vi "test Flush.vi"(8 "error in (no error)":errorcluster, 11 "TestCase in":refnum<class "Message Queue Test Case.lvclass">) -> (0 "error out":errorcluster, 3 "TestCase out":refnum<class "Message Queue Test Case.lvclass">)   [LabVIEW 2017, in "Message Queue Test Case.lvclass"]
uses:
  Message Queue Test Case.lvclass
  Message Queue Test Case.lvclass/Message Queue Test Case.ctl
  Message/Abstract Message/Abstract Message.lvclass
  Message Queue/Abstract Message Queue/Abstract Message Queue.lvclass
  <vilib>/addons/_JKI Toolkits/VI Tester/TestCase.llb/TestCase.lvclass
  C:/Program Files (x86)/National Instruments/LabVIEW 2017/vi.lib/addons/_JKI Toolkits/VI Tester/TestCase.llb/TestCase.lvclass
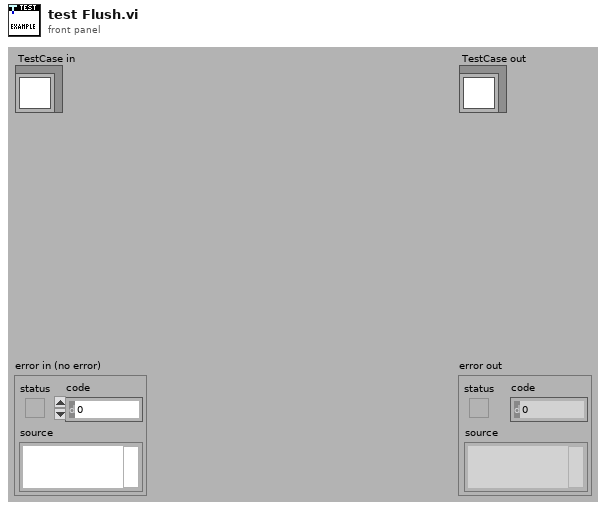
[diagram p1: front panel]
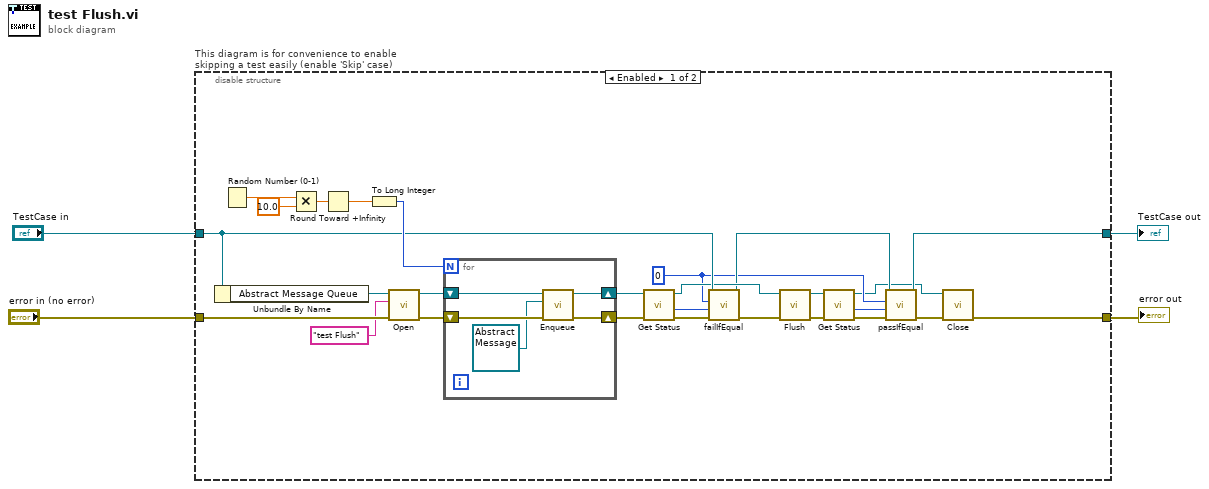
[diagram p0: block diagram]
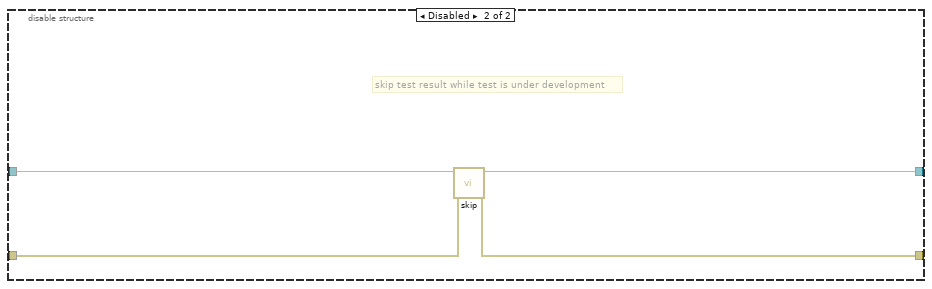
[diagram p2: hidden frame]
diagram:
  n1 = disable-structure "This diagram is for convenience to enable skipping a test easily (enable 'Skip' case)" shown="Enabled" {
    disable-tunnel: "TestCase in" -> [w21 w40]
    disable-tunnel: [w13 w38] -> w1
    disable-tunnel: [w11 w39] -> w3
    disable-tunnel: "error in (no error)" -> [w31 w37]
    frame Enabled {
      w10 = 0 ("current number of messages")
      n2 = Unbundle By Name(w21) -> ("Abstract Message Queue"=w30:refnum<class "Abstract Message Queue.lvclass">)
      n3 = Random Number (0-1)() -> (number: 0 to 1=w28:dbl)
      n4 = Multiply(x=w28, y=10.0) -> (x*y=w26:dbl)
      n5 = Round Toward +Infinity(x=w26) -> (ceil(x): smallest int >= x=w25:dbl)
      n6 = To Long Integer(number=w25) -> (32bit integer=w24:i32)
      n7 = call-dynamic "Open.vi"("error in (no error)"=w31, "name (unnamed)"="test Flush", "Abstract Message Queue in"=w30) -> ("error out"=w23:errorcluster, "Abstract Message Queue out"=w22:refnum<class "Abstract Message Queue.lvclass">)  [unwired: 7 in]
      n8 = for {
        N: w24 -> [_]
        shift-right: [w33] -> w20
        shift-left: w23 -> [w36]
        shift-right: [w32] -> w19
        shift-left: w22 -> [w35]
        n9 = call-dynamic "Enqueue.vi"("error in (no error)"=w36, "Message in"=refnum<class "Abstract Message.lvclass"> refnum, "Abstract Message Queue in"=w35) -> ("error out"=w33:errorcluster, "Abstract Message Queue out"=w32:refnum<class "Abstract Message Queue.lvclass">)  [unwired: 7 in]
      }
      n10 = call-dynamic "Get Status.vi"("error in (no error)"=w20, "Abstract Message Queue in"=w19) -> ("error out"=w17:errorcluster, "current number of messages"=w18:i32, "Abstract Message Queue out"=w15:refnum<class "Abstract Message Queue.lvclass">)  [unwired: 6 in, 1 out]
      n11 = call-dynamic "failIfEqual.vi"("error in (no error)"=w17, "y"=w18, "x"=w10, "TestCase in"=w21) -> ("error out"=w16:errorcluster, "TestCase out"=w14:refnum<class "Message Queue Test Case.lvclass">)  [unwired: 6 in]
      n12 = call-dynamic "Flush.vi"("error in (no error)"=w16, "Abstract Message Queue in"=w15) -> ("error out"=w9:errorcluster, "Abstract Message Queue out"=w8:refnum<class "Abstract Message Queue.lvclass">)  [unwired: 8 in]
      n13 = call-dynamic "Get Status.vi"("error in (no error)"=w9, "Abstract Message Queue in"=w8) -> ("error out"=w7:errorcluster, "current number of messages"=w5:i32, "Abstract Message Queue out"=w6:refnum<class "Abstract Message Queue.lvclass">)  [unwired: 6 in, 1 out]
      n14 = call-dynamic "passIfEqual.vi"("error in (no error)"=w7, "y"=w5, "x"=w10, "TestCase in"=w14) -> ("error out"=w12:errorcluster, "TestCase out"=w13:refnum<class "Message Queue Test Case.lvclass">)  [unwired: 6 in]
      n15 = call-dynamic "Close.vi"("error in (no error)"=w12, "Abstract Message Queue in"=w6) -> ("error out"=w11:errorcluster)  [unwired: 8 in, 1 out]
    }
    frame Disabled {
      # "skip test result while test is under development"
      n16 = call <vilib>:"skip.vi"("error in (no error)"=w37, "TestCase in"=w40) -> ("error out"=w39:errorcluster, "TestCase out"=w38:refnum<class "Message Queue Test Case.lvclass">)  [unwired: 8 in]
    }
  }
  "error out" <- w3
  "TestCase out" <- w1
